vi "sub_write_datafile.vi"(8 "error in (no error)":errorcluster, 10 "Dynamic data":T1, 11 "Input parameters":T2={"Measurement type"=enum."Debug", "Sensor type"=enum."HPK_8in_256ch", "Identifier"="test.txt", "Open after execution?"=FALSE, "Plot after execution?"=FALSE, "Display channel"=0, "Voltage Delay (s)"=0.5, "Switch Delay (s)"=0.01, "VISA resource name source"="", "VISA resource name DMM"="", "VISA resource name LCR"="", "Compliance  Level (A)"=10.0, "Voltage Limit (V)"=1000.0, "Data storage location"="", "Scan voltages"="", "Use source as DMM?"=FALSE, "LCR signal frequenzy (Hz)"=10.0, "DMM device"=enum."Keithley2001", "Sampling number"=1, "Use env. sensors on"=enum."Sensirion sht1x/7x", "Switchboard Handle"=0, "Use Switchboard"=FALSE, "LCR signal voltage (V)"=10000.0, "Repeat"=1, "Scan voltages IV"="", "Scan voltages CV"="", "Hex pad numbers?"=FALSE, "Set measurement type"=enum."Debug", "Custom pad scan"="", "IV voltage Delay (s)"=0.5, "CV voltage Delay (s)"=0.5, "Needle measurement?"=FALSE, "Comments"="test.txt", "LCR signal frequenzy (kHz)"=10.0, "Compliance  Level (uA)"=10.0, "Open Correction Array"=array2304x3[6912 elements], "Current set voltage"=0.0, "Last set voltage"=0.0, "Current channel"=0, "Last OpenCorrection index"=-1, "Total curr/vltg every x steps"=10, "Current channel iteration"=0, "No CV corrections"=FALSE, "Mapfile"="", "Corrfile"="", "IV voltage file"=path "", "CV voltage file"=path "", "IV Switch Delay (s)"=0.01, "CV Switch Delay (s)"=0.01, "Invert polarity"=FALSE, "Set debug dirs"=FALSE, "Is n on p"=FALSE} {"CV Switch Delay (s)" format="%#_13g"; "IV Switch Delay (s)" format="%#_13g"; "Last set voltage" format="%#_13g"; "Current set voltage" format="%#_13g"; "CV voltage Delay (s)" format="%#_13g"; "IV voltage Delay (s)" format="%#_13g"; "Voltage Limit (V)" format="%#_13g"; "Voltage Delay (s)" format="%#_13g"; "Switch Delay (s)" format="%#_13g"}) -> (0 "error out":errorcluster, 2 "Text":string)   [LabVIEW 2016]
doc: "Writes the user input and recorded data to disk."
uses:
  input_params.ctl
  data_dynamic.ctl
  <vilib>/Utility/file.llb/Write Delimited Spreadsheet (string).vi
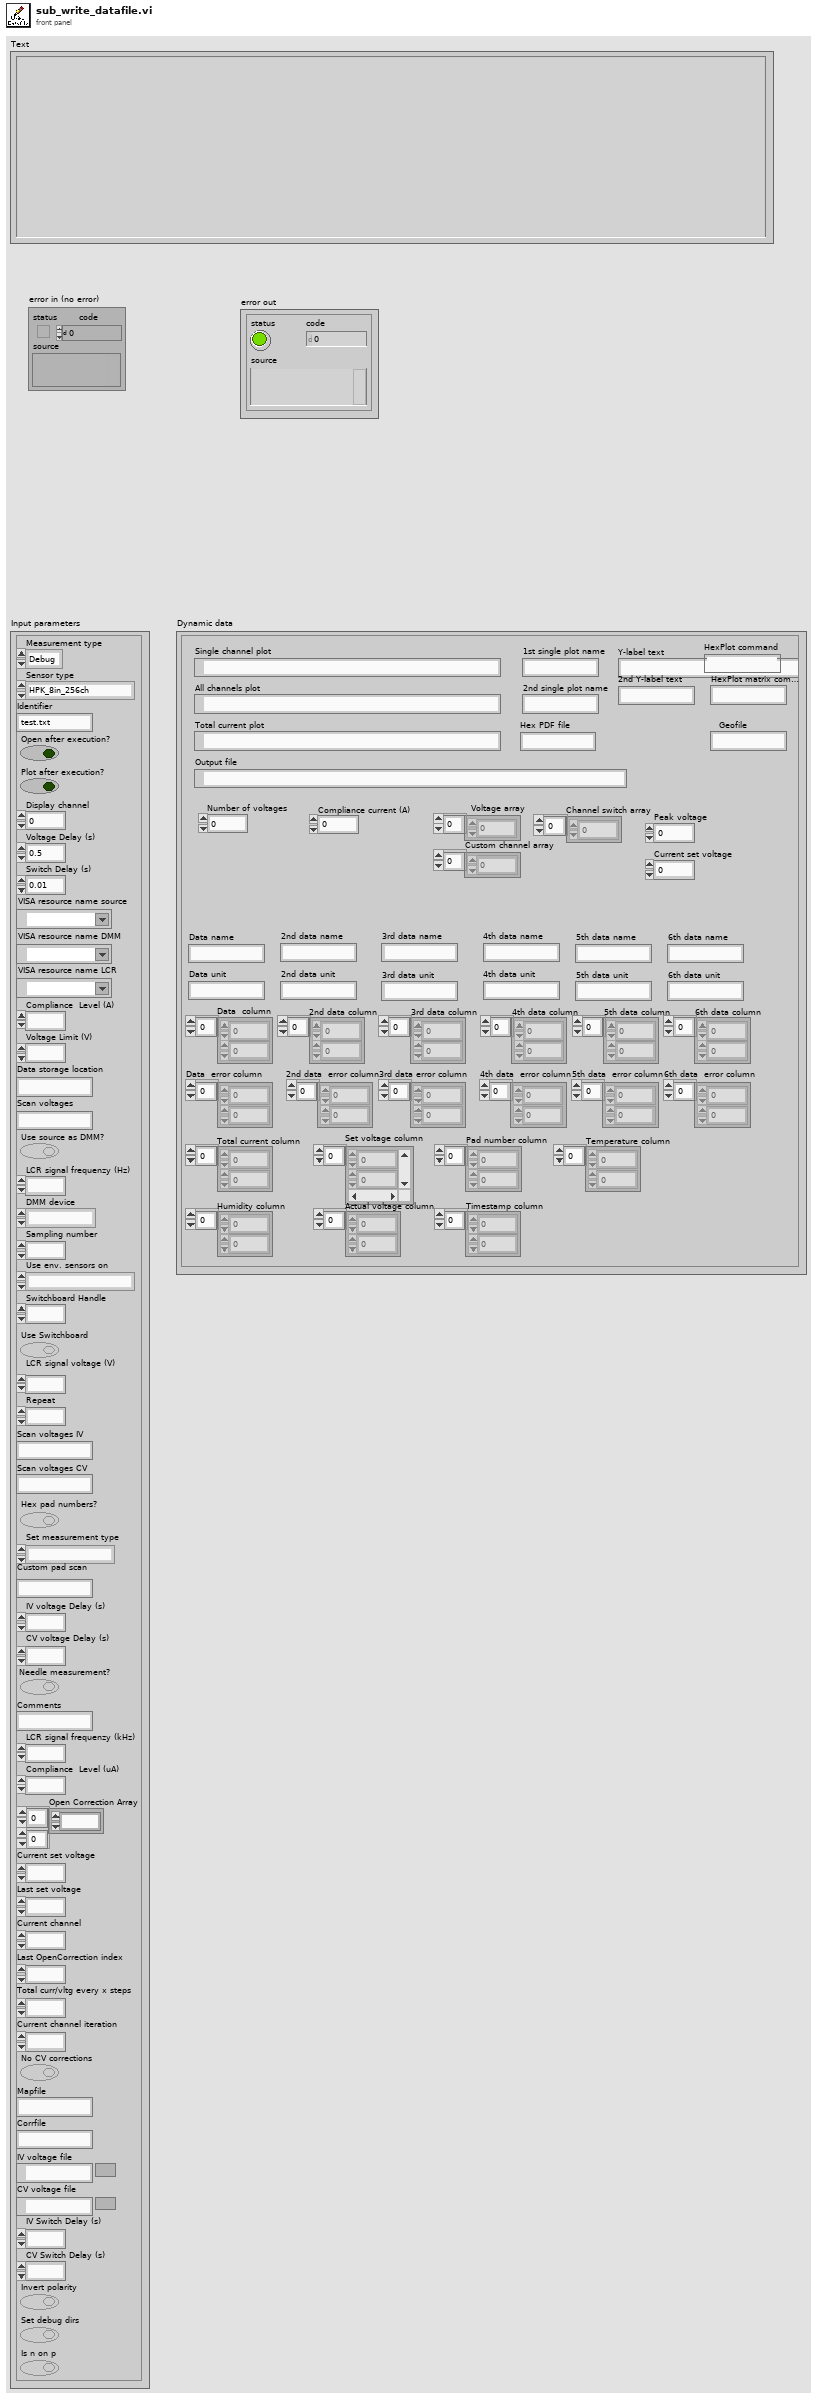
[diagram p1: front panel]
types:
  T1 = typedef "data_dynamic.ctl" = cluster{"Output file":path, "Y-label text":string, "Current set voltage":dbl, "Set voltage column":dbl[], "Pad number column":dbl[], "Data  column":dbl[], "Number of voltages":i32, "Compliance current (A)":dbl, "Geofile":string, "Peak voltage":dbl, "Hex PDF file":string, "Voltage array":dbl[], "Total current column":dbl[], "Timestamp column":dbl[], "Data name":string, "Data unit":string, "2nd data column":dbl[], "2nd data name":string, "2nd data unit":string, "3rd data column":dbl[], "4th data column":dbl[], "3rd data name":string, "3rd data unit":string, "4th data name":string, "4th data unit":string, "Actual voltage column":dbl[], "2nd Y-label text":string, "Single channel plot":path, "Temperature column":dbl[], "Humidity column":dbl[], "Channel switch array":i32[], "1st single plot name":string, "2nd single plot name":string, "All channels plot":path, "HexPlot command":string, "Custom channel array":i32[], "Data  error column":dbl[], "2nd data  error column":dbl[], "3rd data error column":dbl[], "4th data  error column":dbl[], "Total current plot":path, "5th data column":dbl[], "5th data  error column":dbl[], "6th data column":dbl[], "6th data  error column":dbl[], "5th data name":string, "5th data unit":string, "6th data name":string, "6th data unit":string, "HexPlot matrix command":string}
  T2 = typedef "input_params.ctl" = cluster{"Measurement type":enum16{"IV", "CV", "Debug", "Test_contact"}, "Sensor type":enum16{"HPK_6in_135ch", "HPK_8in_256ch", "IFX_8in_256ch", "Diode", "HPK_6in_256ch", "Full_Matrix", ""}, "Identifier":string, "Open after execution?":bool, "Plot after execution?":bool, "Display channel":i32, "Voltage Delay (s)":dbl, "Switch Delay (s)":dbl, "VISA resource name source":refnum<visa-resource-name>, "VISA resource name DMM":refnum<visa-resource-name>, "VISA resource name LCR":refnum<visa-resource-name>, "Compliance  Level (A)":dbl, "Voltage Limit (V)":dbl, "Data storage location":string, "Scan voltages":string, "Use source as DMM?":bool, "LCR signal frequenzy (Hz)":dbl, "DMM device":enum16{"Keithley2001", "Keithley2450", "Keithley2410", "Keithley6487"}, "Sampling number":i32, "Use env. sensors on":enum16{"Sensirion sht1x/7x", "Switch Matrix", "Probecard"}, "Switchboard Handle":u32, "Use Switchboard":bool, "LCR signal voltage (V)":dbl, "Repeat":i32, "Scan voltages IV":string, "Scan voltages CV":string, "Hex pad numbers?":bool, "Set measurement type":enum16{"IV", "CV", "Debug", "Test_contact", "IV+CV"}, "Custom pad scan":string, "IV voltage Delay (s)":dbl, "CV voltage Delay (s)":dbl, "Needle measurement?":bool, "Comments":string, "LCR signal frequenzy (kHz)":dbl, "Compliance  Level (uA)":dbl, "Open Correction Array":dbl[][], "Current set voltage":dbl, "Last set voltage":dbl, "Current channel":i32, "Last OpenCorrection index":i32, "Total curr/vltg every x steps":i32, "Current channel iteration":i32, "No CV corrections":bool, "Mapfile":string, "Corrfile":string, "IV voltage file":path, "CV voltage file":path, "IV Switch Delay (s)":dbl, "CV Switch Delay (s)":dbl, "Invert polarity":bool, "Set debug dirs":bool, "Is n on p":bool}
  T3 = enum16{"HPK_6in_135ch", "HPK_8in_256ch", "IFX_8in_256ch", "Diode", "HPK_6in_256ch", "Full_Matrix", ""}
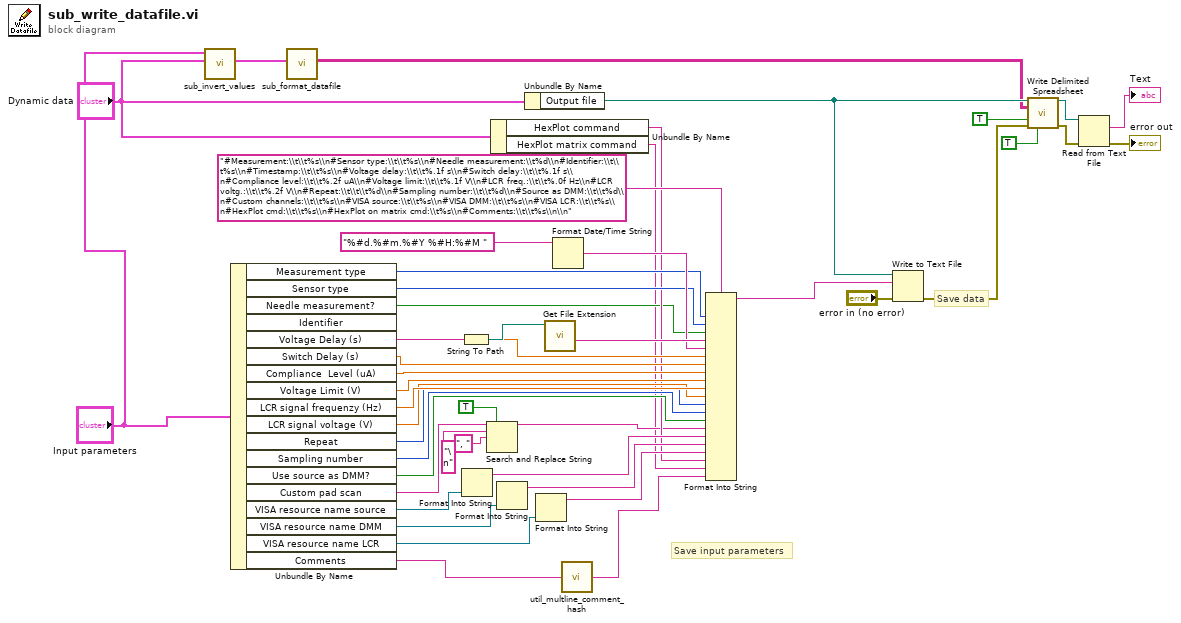
[diagram p0: block diagram]
diagram:
  # "Save data"
  # "Save input parameters"
  n1 = call "sub_invert_values.vi"("Dynamic data"="Dynamic data", "Input parameters"="Input parameters") -> ("Dynamic data out"=w1:T1)  [unwired: 9 in]
  n2 = Unbundle By Name("Input parameters") -> ("Measurement type"=w40:enum16{"IV", "CV", "Debug", "Test_contact"}, "Sensor type"=w39:T3, "Needle measurement?"=w8:bool, "Identifier"=w38:string, "Voltage Delay (s)"=w37:dbl, "Switch Delay (s)"=w36:dbl, "Compliance  Level (uA)"=w35:dbl, "Voltage Limit (V)"=w34:dbl, "LCR signal frequenzy (Hz)"=w32:dbl, "LCR signal voltage (V)"=w31:dbl, "Repeat"=w29:i32, "Sampling number"=w30:i32, "Use source as DMM?"=w33:bool, "Custom pad scan"=w11:string, "VISA resource name source"=w28:refnum<visa-resource-name>, "VISA resource name DMM"=w27:refnum<visa-resource-name>, "VISA resource name LCR"=w26:refnum<visa-resource-name>, "Comments"=w6:string)
  n3 = call "sub_format_datafile.vi"("Dynamic data"=w1) -> ("appended array"=w4:string[][])  [unwired: 10 in]
  n4 = String To Path(string=w38) -> (path=w45:path)
  n5 = Format Into String(w28) -> (resulting string=w25:string)  [unwired: 3 in, 1 out]
  n6 = Search and Replace String(replace all?=TRUE ("replace all? (F)"), input string=w11, search string="\n", replace string=", " ("replace string (\"\")")) -> (result string=w10:string)  [unwired: 4 in, 3 out]
  n7 = Unbundle By Name("Dynamic data") -> ("HexPlot command"=w14:string, "HexPlot matrix command"=w7:string)
  n8 = Format Into String(w27) -> (resulting string=w24:string)  [unwired: 3 in, 1 out]
  n9 = Unbundle By Name("Dynamic data") -> ("Output file"=w20:path)
  n10 = Format Into String(w26) -> (resulting string=w23:string)  [unwired: 3 in, 1 out]
  n11 = call <vilib>:"Get File Extension.vi"("file"=w45) -> ("filename without extension"=w44:string)  [unwired: 6 in, 4 out]
  n12 = Format Date/Time String(time format string (%c)="%#d.%#m.%#Y %#H:%#M ") -> (date/time string=w42:string)  [unwired: 2 in]
  n13 = call "util_multline_comment_hash.vi"("input string"=w6) -> ("result string"=w5:string)
  n14 = Format Into String(format string="#Measurement:\\t\\t%s\\n#Sensor type:\\t\\t%s\\n#Needle measurement:\\t%d\\n#Identifier:\\t\\t%s\\n#Timestamp:\\t\\t%s\\n#Voltage delay:\\t\\t%.1f s\\n#Switch delay:\\t\\t%.1f s\\n#Compliance level:\\t\\t%.2f uA\\n#Voltage limit:\\t\\t%.1f V\\n#LCR freq.:\\t\\t%.0f Hz\\n#LCR voltg.:\\t\\t%.2f V\\n#Repeat:\\t\\t\\t%d\\n#Sampling number:\\t\\t%d\\n#Source as DMM:\\t\\t%d\\n#Custom channels:\\t\\t%s\\n#VISA source:\\t\\t%s\\n#VISA DMM:\\t\\t%s\\n#VISA LCR:\\t\\t%s\\n#HexPlot cmd:\\t\\t%s\\n#HexPlot on matrix cmd:\\t%s\\n#Comments:\\t\\t%s\\n\\n", w40, w39, w8, w44, w42, w37, w36, w35, w34, w32, w31, w29, w30, w33, w10, w25, w24, w23, w14, w7, w5) -> (resulting string=w46:string)  [unwired: 2 in, 1 out]
  n15 = Write to Text File(file (use dialog)=w20, text=w46, error in="error in (no error)") -> (error out=w19:errorcluster)  [unwired: 1 in, 2 out]
  n16 = call-poly <vilib>:"Write Delimited Spreadsheet.vi"("file path (dialog if empty)"=w20, "2D data"=w4, "append to file? (new file:F)"=TRUE, "error in (no error)"=w19, "transpose? (no:F)"=TRUE) -> ("new file path (Not A Path if cancelled)"=w16:path, "error out"=w18:errorcluster)  [unwired: 9 in]
  n17 = Read from Text File(file (use dialog)=w16, error in=w18) -> (text=→"Text":string, error out=→"error out":errorcluster)  [unwired: 2 in, 2 out]
